vi "S8300E_SetTP_Temperature_CriteriaTOOL.vi"() -> ()   [LabVIEW 2011]
panel:
  in  "Tab Control":enum32{"Page 1"}(tab)
  in  "MB High Limit(C)":dbl format="%#.6f"
  in  "MB Lower Limit (C":dbl format="%#.6f"
  out "TestPoint_Name 6":string="TP46"
  in  "DDR3 Slot2  High Limit(C)":dbl format="%#.6f"
  in  "DDR3 Slot2 Lower Limit (C)":dbl format="%#.6f"
  out "TestPoint_Name 4":string="TP46"
  in  "DDR3 Slot1 High Limit(C)":dbl format="%#.6f"
  in  "DDR3 Slot1 Lower Limit (C)":dbl format="%#.6f"
  out "TestPoint_Name 3":string="TP46"
  in  "PCH High Limit(C)":dbl format="%#.6f"
  in  "PCH Lower Limit (C)":dbl format="%#.6f"
  out "TestPoint_Name 2":string="TP46"
  in  "High Limit Temperature":dbl format="%#.6f"
  in  "Lower Limit Temperature":dbl format="%#.6f"
  out "TestPoint_Name":string="TP46"
  out "TestPoint_Name 5":string="TP46"
  in  "CPU2 Lower Limit Temperature":dbl format="%#.6f"
  in  "CPU2 High Limit Temperature":dbl format="%#.6f"
  out "DatalogType":T1(array[cluster]) {"Lower Limit Voltage" format="%#.6f"; "High Limit Voltage" format="%#.6f"}
  in  "儲存離開":bool
  # "2014-8-6"
  # "S8300E Temperature Test Point Criteria Setting\nS8300E 各測點溫度 設定"
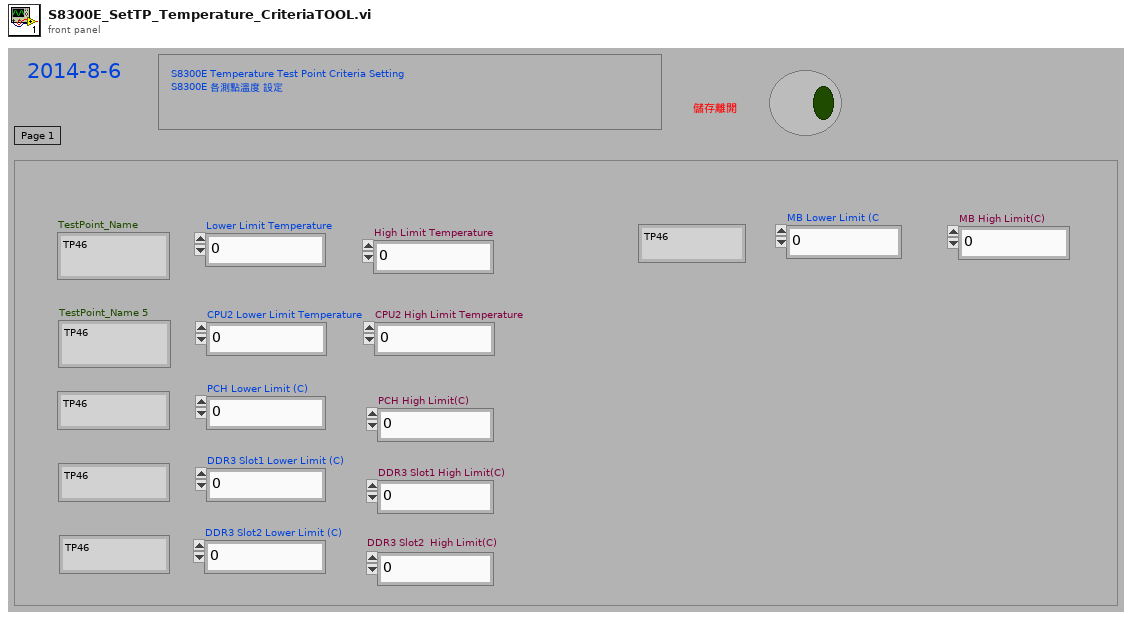
[diagram p1: front panel]
types:
  T1 = cluster{"TestPoint_Name":string, "Lower Limit Voltage":dbl, "High Limit Voltage":dbl, cluster{"Relay3 Name":string, "Relay3H/L":bool}[], "Measure Ai name":string}[]
  T2 = enum16{"open", "replace", "create", "open or create", "replace or create", "replace or create with confirmation"}
  T3 = cluster{"TestPoint_Name":string, "Lower Limit Voltage":dbl, "High Limit Voltage":dbl, cluster{"Relay3 Name":string, "Relay3H/L":bool}[], "Measure Ai name":string}
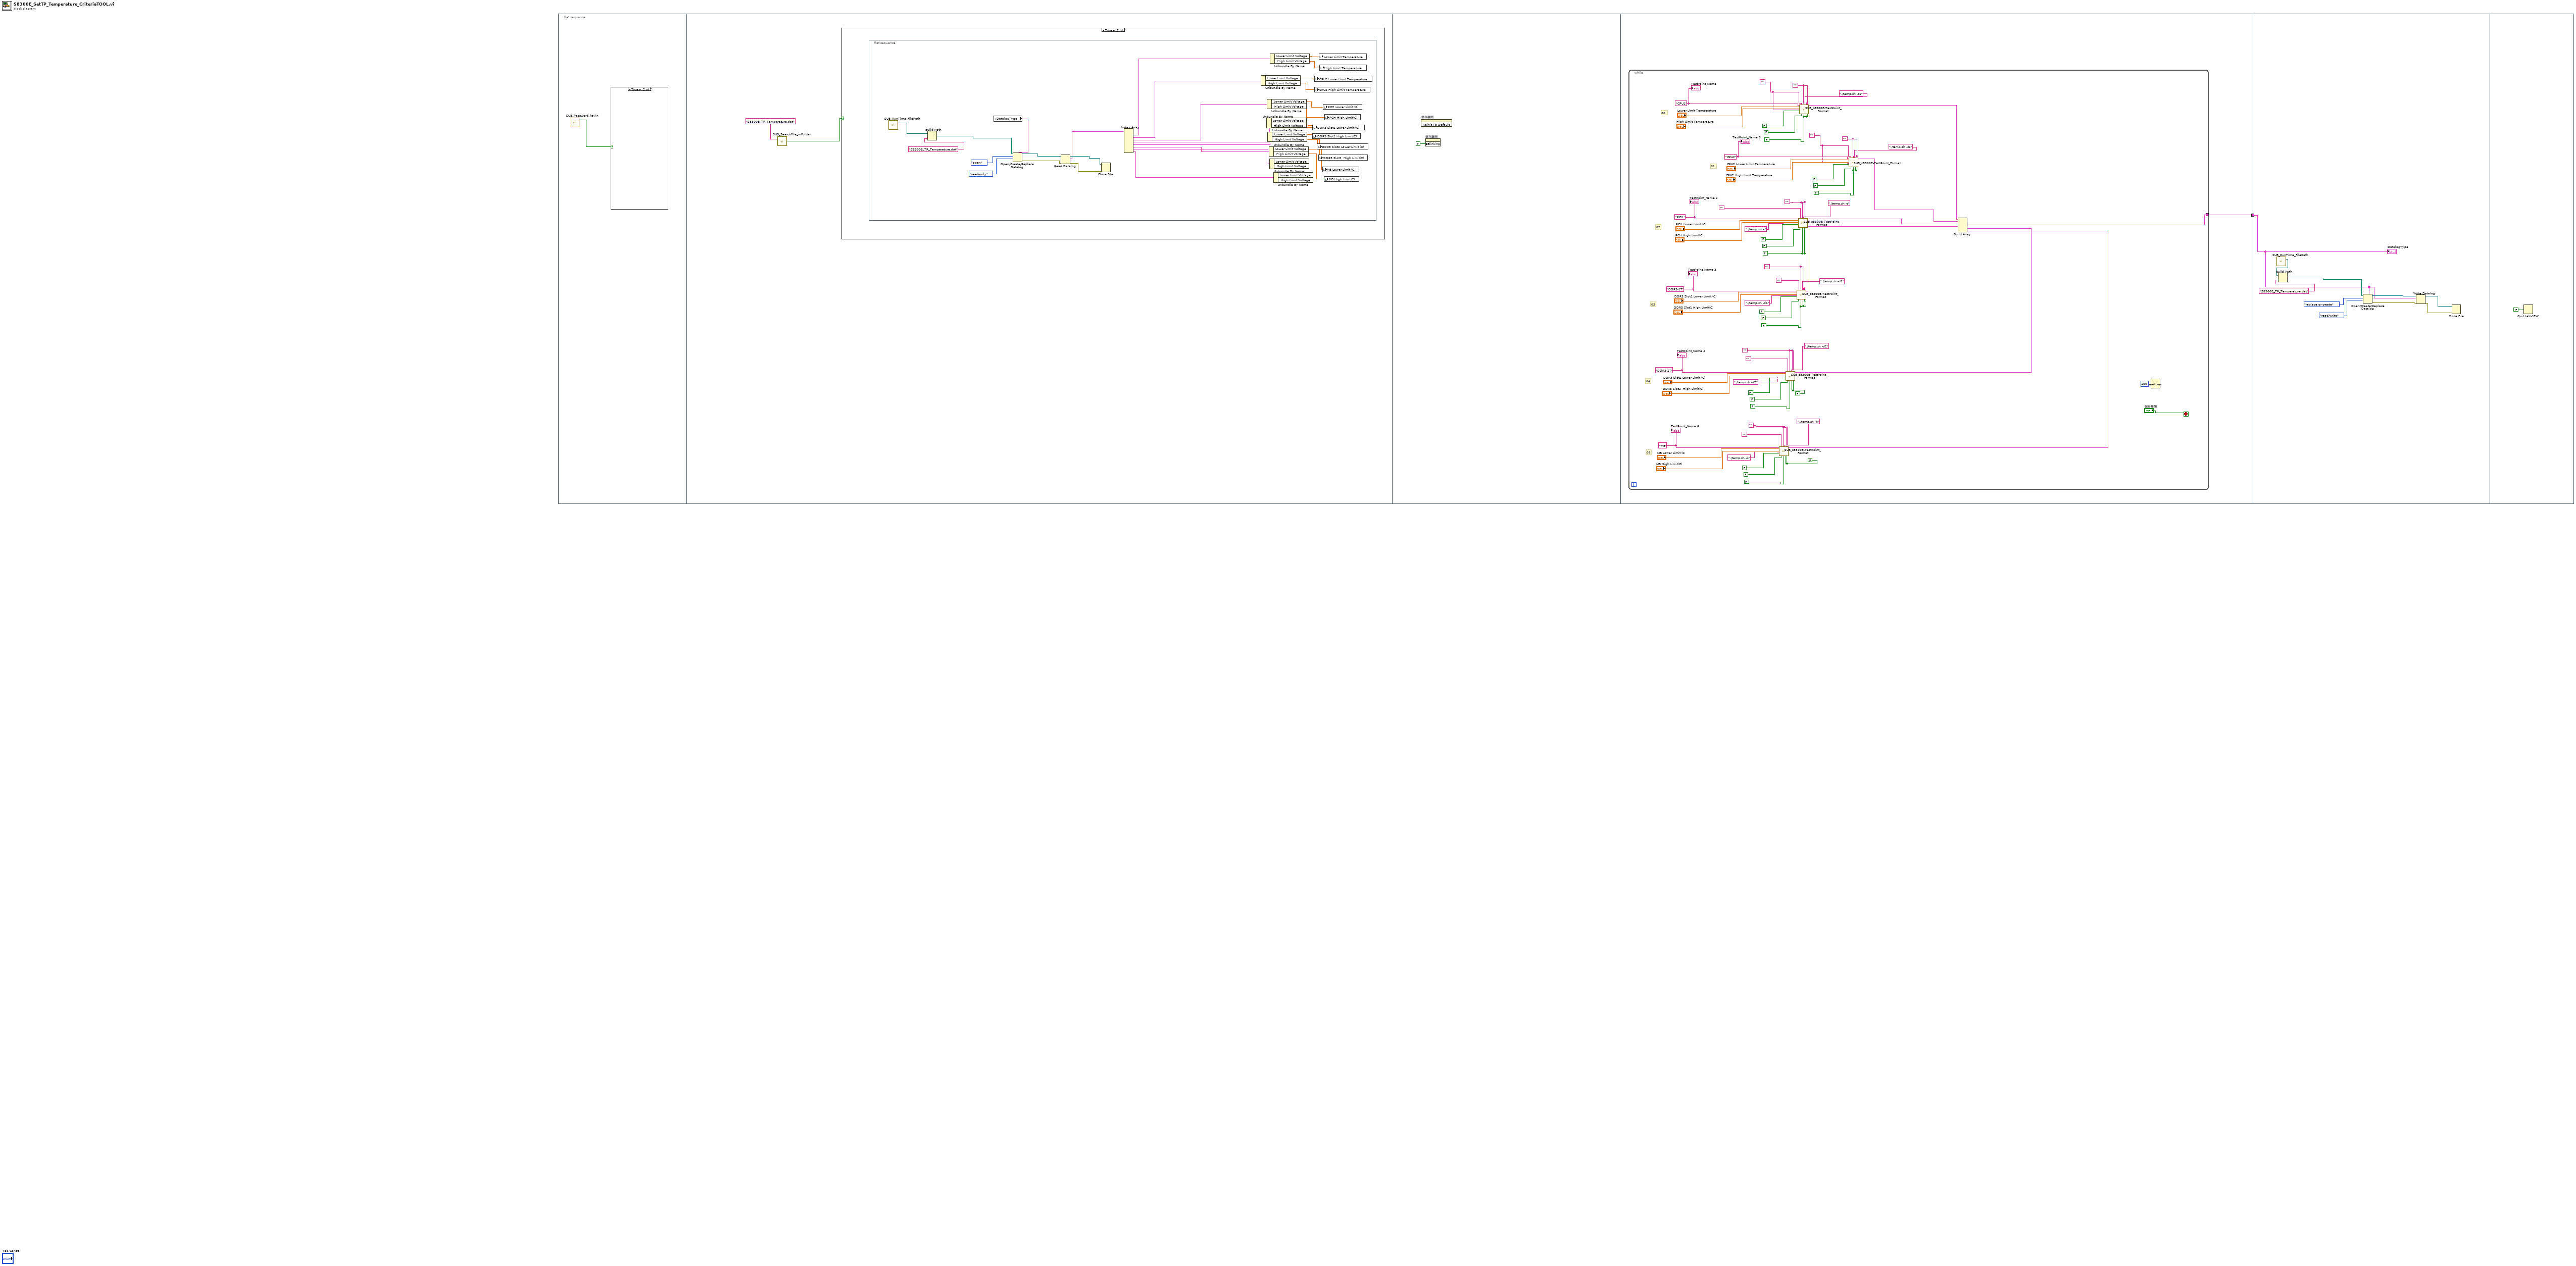
[diagram p0: block diagram]
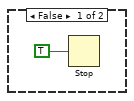
[diagram p2: hidden frame]
diagram:
  n1 = flat-sequence {
    tunnel: [w38] -> w1
    tunnel: w1 -> [w108]
    frame #0 {
      n2 = call "SUB_Password_keyin.vi"() -> ("Pass?"=w2:bool)  [unwired: 3 in]
      n3 = case shown="True" w2 {
        frame False {
          n4 = Stop(stop? (T)=TRUE) -> ()
        }
        frame True {
        }
      }
    }
    frame #1 {
      n5 = call "SUB_SearchFile_inFolder.vi"("Search Filename in Folder"="S8300E_TP_Temperature.dat" ("name or relative path")) -> ("File Existing True/Flase"=w4:bool)  [unwired: 1 in]
      n6 = case shown="True" w4 {
        frame False {
        }
        frame True {
          n7 = flat-sequence {
            frame #0 {
              n8 = call "SUB_RunTime_FilePath.vi"() -> ("stripped path"=w28:path)  [unwired: 3 in]
              n9 = Build Path(base path=w28, name or relative path="S8300E_TP_Temperature.dat") -> (appended path=w33:path)
              n10 = local read "DatalogType"() -> (w27:T1)
              n11 = Open/Create/Replace Datalog(5:w27, 9:enum16{"read/write", "read-only", "write-only"}."read-only" ("access (0:read/write)"), 10:T2."open" ("operation (0:open)"), 11:w33) -> (0:w30:errorcluster, 3:w29:refnum<k1>)  [unwired: 2 in, 1 out]
              n12 = Read Datalog(4:w30, 7:w29) -> (0:w32:errorcluster, 2:w26:T1, 3:w31:refnum<k1>)  [unwired: 1 in]
              n13 = Close File(refnum=w31, error in=w32) -> ()  [unwired: 2 out]
              n14 = Index Array(array=w26) -> (element #1=w9:T3, element #2=w8:T3, element #3=w23:T3, element #4=w20:T3, element #5=w17:T3, element #6=w14:T3, element #7=w11:T3, element #8=w10:T3)  [unwired: 8 in]
              n15 = Unbundle By Name(w8) -> ("Lower Limit Voltage"=w7:dbl, "High Limit Voltage"=w6:dbl)
              n16 = Unbundle By Name(w20) -> ("Lower Limit Voltage"=w19:dbl, "High Limit Voltage"=w18:dbl)
              n17 = Unbundle By Name(w23) -> ("Lower Limit Voltage"=w22:dbl, "High Limit Voltage"=w21:dbl)
              n18 = Unbundle By Name(w17) -> ("Lower Limit Voltage"=w16:dbl, "High Limit Voltage"=w15:dbl)
              n19 = Unbundle By Name(w14) -> ("Lower Limit Voltage"=w13:dbl, "High Limit Voltage"=w12:dbl)
              n20 = Unbundle By Name(w11) -> ()  [unwired: 2 out]
              n21 = Unbundle By Name(w9) -> ("Lower Limit Voltage"=w25:dbl, "High Limit Voltage"=w24:dbl)
              n22 = Unbundle By Name(w10) -> ()  [unwired: 2 out]
              n23 = local write "DDR3 Slot1 High Limit(C)"(w18) -> ()
              n24 = local write "DDR3 Slot1 Lower Limit (C)"(w19) -> ()
              n25 = local write "CPU2 Lower Limit Temperature"(w7) -> ()
              n26 = local write "CPU2 High Limit Temperature"(w6) -> ()
              n27 = local write "DDR3 Slot2 Lower Limit (C)"(w16) -> ()
              n28 = local write "DDR3 Slot2  High Limit(C)"(w15) -> ()
              n29 = local write "Lower Limit Temperature"(w25) -> ()
              n30 = local write "High Limit Temperature"(w24) -> ()
              n31 = local write "MB Lower Limit (C"(w13) -> ()
              n32 = local write "PCH Lower Limit (C)"(w22) -> ()
              n33 = local write "MB High Limit(C)"(w12) -> ()
              n34 = local write "PCH High Limit(C)"(w21) -> ()
            }
          }
        }
      }
    }
    frame #2 {
      n35 = invoke on="儲存離開" class="Bool (strict)" method="Reinit To Default"() -> ()  [unwired: 3 in, 3 out]
      n36 = property on="儲存離開" class="Bool (strict)"("Blinking"=TRUE) -> ()  [unwired: 2 in, 2 out]
    }
    frame #3 {
      n37 = while {
        tunnel: [w61] -> w38
        stop <- "儲存離開" stop-if-true
        w41 = ""
        w42 = ""
        w43 = FALSE
        w48 = "CPU2" ("TestPoint_Name")
        w50 = ""
        w67 = FALSE
        w68 = ""
        w69 = FALSE
        w70 = ""
        w72 = ""
        w74 = ""
        w59 = ""
        w83 = "MB" ("TestPoint_Name")
        w90 = "DDR3-2T" ("TestPoint_Name")
        w71 = FALSE
        w96 = "DDR3-1T" ("TestPoint_Name")
        w73 = FALSE
        w102 = "PCH " ("TestPoint_Name")
        w75 = FALSE
        w107 = "CPU1" ("TestPoint_Name")
        # "01"
        # "05"
        # "04"
        # "03"
        # "02"
        # "00"
        n38 = call "SUB_s8300E-TestPoint_Format.vi"("TestPoint_Name"=w83, "Lower Limit Voltage"="MB Lower Limit (C", "High Limit Voltage"="MB High Limit(C)", "Relay 1 Name"="./temp.sh -b", "Relay1 H/L"=FALSE, "Relay 2 Name"="", "Relay2 H/L"=FALSE, "Relay3 Name"=w68, "Relay3H/L"=FALSE, "Measure Ai name"="./temp.sh -b", "Relay4 Name"=w68, "Relay4 H/L"=w67, "Relay5 Name"=w68, "Relay5 H/L"=w67) -> ("output cluster"=w62:T3)  [unwired: 13 in]
        n39 = call "SUB_s8300E-TestPoint_Format.vi"("TestPoint_Name"=w90, "Lower Limit Voltage"="DDR3 Slot2 Lower Limit (C)", "High Limit Voltage"="DDR3 Slot2  High Limit(C)", "Relay 1 Name"="./temp.sh -d2", "Relay1 H/L"=FALSE, "Relay 2 Name"="", "Relay2 H/L"=FALSE, "Relay3 Name"=w70, "Relay3H/L"=FALSE, "Measure Ai name"="./temp.sh -d2", "Relay4 Name"=w70, "Relay4 H/L"=w69, "Relay5 Name"=w70, "Relay5 H/L"=w69) -> ("output cluster"=w63:T3)  [unwired: 13 in]
        n40 = call "SUB_s8300E-TestPoint_Format.vi"("TestPoint_Name"=w96, "Lower Limit Voltage"="DDR3 Slot1 Lower Limit (C)", "High Limit Voltage"="DDR3 Slot1 High Limit(C)", "Relay 1 Name"="./temp.sh -d1", "Relay1 H/L"=FALSE, "Relay 2 Name"="", "Relay2 H/L"=FALSE, "Relay3 Name"=w72, "Relay3H/L"=w71, "Measure Ai name"="./temp.sh -d1", "Relay4 Name"=w72, "Relay4 H/L"=w71, "Relay5 Name"=w72, "Relay5 H/L"=w71) -> ("output cluster"=w64:T3)  [unwired: 13 in]
        n41 = call "SUB_s8300E-TestPoint_Format.vi"("TestPoint_Name"=w102, "Lower Limit Voltage"="PCH Lower Limit (C)", "High Limit Voltage"="PCH High Limit(C)", "Relay 1 Name"="./temp.sh -s", "Relay1 H/L"=FALSE, "Relay 2 Name"="", "Relay2 H/L"=FALSE, "Relay3 Name"=w74, "Relay3H/L"=w73, "Measure Ai name"="./temp.sh -s", "Relay4 Name"=w74, "Relay4 H/L"=w73, "Relay5 Name"=w74, "Relay5 H/L"=w73) -> ("output cluster"=w65:T3)  [unwired: 13 in]
        n42 = call "SUB_s8300E-TestPoint_Format.vi"("TestPoint_Name"=w107, "Lower Limit Voltage"="Lower Limit Temperature", "High Limit Voltage"="High Limit Temperature", "Relay 1 Name"=w50, "Relay1 H/L"=FALSE, "Relay 2 Name"=w50, "Relay2 H/L"=FALSE, "Relay3 Name"=w59, "Relay3H/L"=w75, "Measure Ai name"="./temp.sh -c1", "Relay4 Name"=w59, "Relay4 H/L"=w75, "Relay5 Name"=w59, "Relay5 H/L"=w75) -> ("output cluster"=w66:T3)  [unwired: 13 in]
        n43 = call "SUB_s8300E-TestPoint_Format.vi"("TestPoint_Name"=w48, "Lower Limit Voltage"="CPU2 Lower Limit Temperature", "High Limit Voltage"="CPU2 High Limit Temperature", "Relay 1 Name"=w41, "Relay1 H/L"=FALSE, "Relay 2 Name"=w41, "Relay2 H/L"=FALSE, "Relay3 Name"=w42, "Relay3H/L"=w43, "Measure Ai name"="./temp.sh -c2", "Relay4 Name"=w42, "Relay4 H/L"=w43, "Relay5 Name"=w42, "Relay5 H/L"=w43) -> ("output cluster"=w39:T3)  [unwired: 13 in]
        n44 = Build Array "Build Array"(w66, w39, w65, w64, w63, w62) -> (w61:T1)
        n45 = Wait (ms)(milliseconds to wait=u32 100) -> ()  [unwired: 1 out]
        "TestPoint_Name" <- w107
        "TestPoint_Name 2" <- w102
        "TestPoint_Name 3" <- w96
        "TestPoint_Name 4" <- w90
        "TestPoint_Name 6" <- w83
        "TestPoint_Name 5" <- w48
      }
    }
    frame #4 {
      n46 = call "SUB_RunTime_FilePath.vi"() -> ("stripped path"=w110:path)  [unwired: 3 in]
      n47 = Build Path(base path=w110, name or relative path="S8300E_TP_Temperature.dat") -> (appended path=w111:path)
      n48 = Open/Create/Replace Datalog(5:w108, 9:enum16{"read/write", "read-only", "write-only"}."read/write" ("access (0:read/write)"), 10:T2."replace or create" ("operation (0:open)"), 11:w111) -> (0:w116:errorcluster, 3:w109:refnum<k1>)  [unwired: 2 in, 1 out]
      n49 = Write Datalog(4:w116, 6:w108, 7:w109) -> (0:w114:errorcluster, 3:w115:refnum<k1>)
      n50 = Close File(refnum=w115, error in=w114) -> ()  [unwired: 2 out]
      "DatalogType" <- w108
    }
    frame #5 {
      n51 = Quit LabVIEW(quit? (T)=FALSE) -> ()
    }
  }
